vi "reentr.vi"() -> ()   [LabVIEW 2017]
panel:
  out "4":dbl
  out "3":dbl
  out "2":dbl
  out "1":dbl
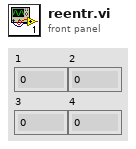
[diagram p1: front panel]
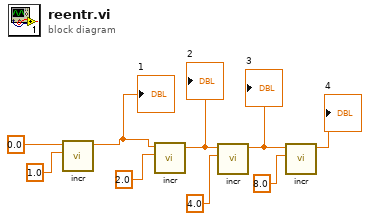
[diagram p0: block diagram]
diagram:
  n1 = call "incr.vi"("y"=1.0, "x"=0.0) -> ("x+1"=w8:dbl)  [unwired: 9 in]
  "1" <- w8
  n2 = call "incr.vi"("y"=2.0, "x"=w8) -> ("x+1"=w7:dbl)  [unwired: 9 in]
  "2" <- w7
  n3 = call "incr.vi"("y"=4.0, "x"=w7) -> ("x+1"=w6:dbl)  [unwired: 9 in]
  "3" <- w6
  n4 = call "incr.vi"("y"=8.0, "x"=w6) -> ("x+1"=→"4":dbl)  [unwired: 9 in]
